vi "iRobot Navigation Display Sensors.vi"(6 "Left Wheel (mm/s)":i16, 7 "Right Wheel (mm/s)":i16, 9 "Statechart Inputs":T1={"net distance (mm)"=0, "net angle (deg)"=0, "Max Wheel Speed (mm/s)"=0, "accelerometer"={"x axis (g)"=0.0, "y axis (g)"=0.0, "z axis (g)"=0.0}, "iRobot Sensors"={"Bumps + Wheel Drops"={"Wheeldrop Caster"=FALSE, "Wheeldrop Left"=FALSE, "Wheeldrop Right"=FALSE, "Bump Left"=FALSE, "Bump Right"=FALSE}, "Wall"=FALSE, "Cliff Left"=FALSE, "Cliff Front Left"=FALSE, "Cliff Front Right"=FALSE, "Cliff Right"=FALSE, "Virtual Wall"=FALSE, "Low-Side Driver + Wheel Overcurrent"={"Low-Side Driver 0"=FALSE, "Low-Side Driver 1"=FALSE, "Low-Side Driver 2"=FALSE, "Left Wheel"=FALSE, "Right Wheel"=FALSE}, "Infrared"=255, "Buttons"={"Advance"=FALSE, "Play"=FALSE}, "Distance (mm)"=0, "Angle (deg)"=0, "Charging State"=enum."Not Charging", "Voltage (mV)"=0, "Current (mA)"=0, "Battery Temperature (deg C)"=0, "Battery Charge (mAh)"=0, "Battery Capacity (mAh)"=0, "Wall Signal (0-4095)"=0, "Cliff Left Signal (0-4095)"=0, "Cliff Front Left Signal (0-4095)"=0, "Cliff Front Right Signal (0-4095)"=0, "Cliff Right Signal (0-4095)"=0, "Cargo Bay Digital Inputs"={"Digital Input 0"=FALSE, "Digital Input 1"=FALSE, "Digital Input 2"=FALSE, "Digital Input 3"=FALSE, "Device Detect"=FALSE}, "Cargo Bay Analog Signal (0-1023)"=0, "Charging Sources Available"={"Internal Charger"=FALSE, "Home Base"=FALSE}, "OI Mode"=enum."Off", "Song Number"=0, "Song Playing"=FALSE, "Number of Stream Packets"=0, "Requested Velocity (mm/s)"=0, "Requested Radius (mm)"=0, "Requested Right Wheel Velocity (mm/s)"=0, "Requested Left Wheel Velocity (mm/s)"=0}, "Is Simulator?"=FALSE, "Edge Tape Threshold"=0, "Barcode Tape Threshold"=0, "Barcode Time Threshold"=0.0, "Barcode Action Time"=0.0, "Kp Constant"=0.0, "Ki Constant"=0.0, "Kd Constant"=0.0} {"iRobot Sensors"."Infrared" format="%02x"; "accelerometer"."z axis (g)" format="%.3f"; "accelerometer"."y axis (g)" format="%.3f"; "accelerometer"."x axis (g)" format="%.3f"; "Max Wheel Speed (mm/s)" scale=0.0..500.0}) -> (1 "iRobot Sensors (graphical)":T11 {"Right Wheel (mm/s)" scale=-500.0..500.0; "Left Wheel (mm/s)" scale=-500.0..500.0})   [LabVIEW 2015]
uses:
  iRobot Sensors.ctl
  iRobot Navigation State Machine.lvsc/Inputs.ctl
  Accelerometer.ctl
  iRobot/Sensor/Sensor Group 6.ctl
  iRobot/Sensor/Bumps + Wheel Drops.ctl
  iRobot/Sensor/Low-Side Driver + Wheel Overcurrent.ctl
  iRobot/Sensor/Buttons.ctl
  iRobot/Sensor/Charging State.ctl
  iRobot/Sensor/Cargo Bay Digital Inputs.ctl
  iRobot/Sensor/Charging Sources Available.ctl
  iRobot/Sensor/OI Mode.ctl
  iRobot Navigation State Machine.lvsc
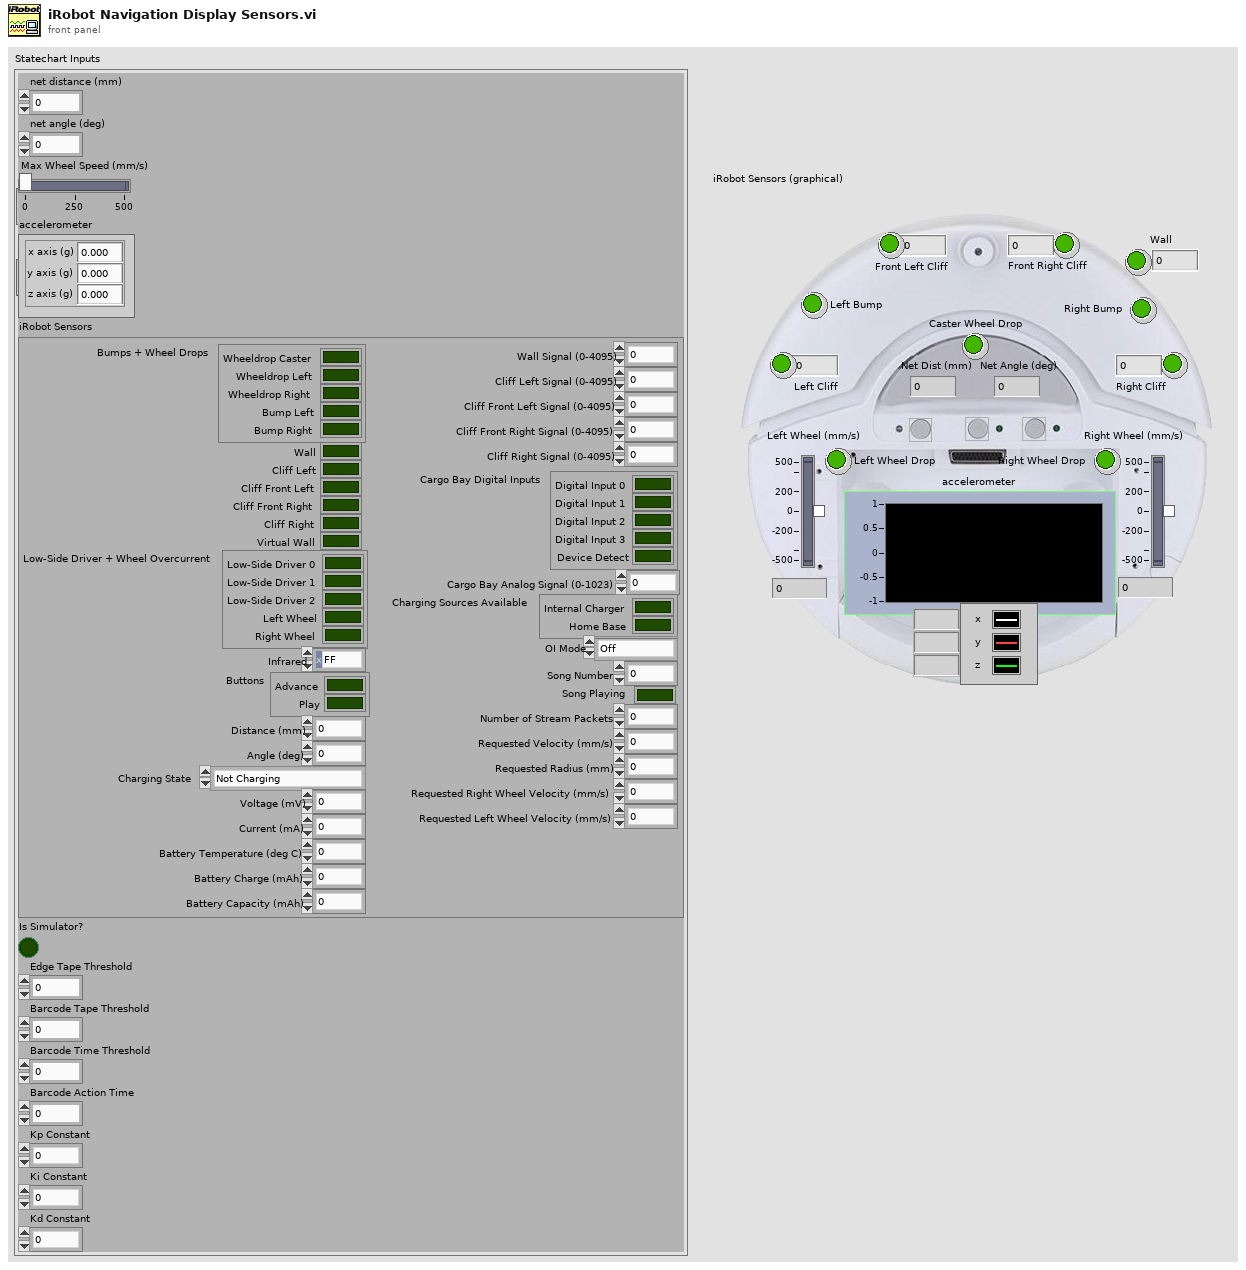
[diagram p1: front panel]
types:
  T1 = typedef "iRobot Navigation State Machine.lvsc/Inputs.ctl" = cluster{"net distance (mm)":i32, "net angle (deg)":i32, "Max Wheel Speed (mm/s)":i16, "accelerometer":T2, "iRobot Sensors":T3, "Is Simulator?":bool, "Edge Tape Threshold":u16, "Barcode Tape Threshold":u16, "Barcode Time Threshold":dbl, "Barcode Action Time":dbl, "Kp Constant":dbl, "Ki Constant":dbl, "Kd Constant":dbl}
  T2 = typedef "Accelerometer.ctl" = cluster{"x axis (g)":dbl, "y axis (g)":dbl, "z axis (g)":dbl}
  T3 = typedef "Sensor Group 6.ctl" = cluster{"Bumps + Wheel Drops":T4, "Wall":bool, "Cliff Left":bool, "Cliff Front Left":bool, "Cliff Front Right":bool, "Cliff Right":bool, "Virtual Wall":bool, "Low-Side Driver + Wheel Overcurrent":T5, "Infrared":u8, "Buttons":T6, "Distance (mm)":i32, "Angle (deg)":i32, "Charging State":T7, "Voltage (mV)":u16, "Current (mA)":i16, "Battery Temperature (deg C)":i8, "Battery Charge (mAh)":u16, "Battery Capacity (mAh)":u16, "Wall Signal (0-4095)":u16, "Cliff Left Signal (0-4095)":u16, "Cliff Front Left Signal (0-4095)":u16, "Cliff Front Right Signal (0-4095)":u16, "Cliff Right Signal (0-4095)":u16, "Cargo Bay Digital Inputs":T8, "Cargo Bay Analog Signal (0-1023)":u16, "Charging Sources Available":T9, "OI Mode":T10, "Song Number":u8, "Song Playing":bool, "Number of Stream Packets":u8, "Requested Velocity (mm/s)":i16, "Requested Radius (mm)":i16, "Requested Right Wheel Velocity (mm/s)":i16, "Requested Left Wheel Velocity (mm/s)":i16}
  T4 = typedef "Bumps + Wheel Drops.ctl" = cluster{"Wheeldrop Caster":bool, "Wheeldrop Left":bool, "Wheeldrop Right":bool, "Bump Left":bool, "Bump Right":bool}
  T5 = typedef "Low-Side Driver + Wheel Overcurrent.ctl" = cluster{"Low-Side Driver 0":bool, "Low-Side Driver 1":bool, "Low-Side Driver 2":bool, "Left Wheel":bool, "Right Wheel":bool}
  T6 = typedef "Buttons.ctl" = cluster{"Advance":bool, "Play":bool}
  T7 = typedef "Charging State.ctl" = enum16{"Not Charging", "Reconditioning Charging", "Full Charging", "Trickle Charging", "Waiting", "Charging Fault Condition"}
  T8 = typedef "Cargo Bay Digital Inputs.ctl" = cluster{"Digital Input 0":bool, "Digital Input 1":bool, "Digital Input 2":bool, "Digital Input 3":bool, "Device Detect":bool}
  T9 = typedef "Charging Sources Available.ctl" = cluster{"Internal Charger":bool, "Home Base":bool}
  T10 = typedef "OI Mode.ctl" = enum16{"Off", "Passive", "Safe", "Full"}
  T11 = typedef "iRobot Sensors.ctl" = cluster{"Caster Wheel Drop":bool, "Left Wheel Drop":bool, "Right Wheel Drop":bool, "Left Bump":bool, "Right Bump":bool, "Left Cliff":bool, "Front Left Cliff":bool, "Front Right Cliff":bool, "Right Cliff":bool, "Wall":bool, "Net Dist (mm)":i32, "Net Angle (deg)":i32, "Wall":u16, "Left Cliff":u16, "Front Left Cliff":u16, "Front Right Cliff":u16, "Right Cliff":u16, "Left Wheel (mm/s)":i16, "Right Wheel (mm/s)":i16, "accelerometer":T2}
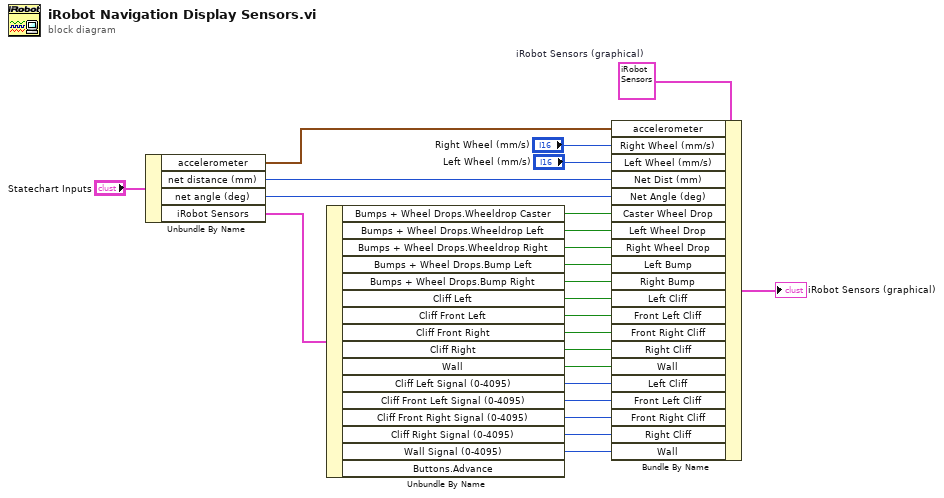
[diagram p0: block diagram]
diagram:
  w7 = T11 {"Caster Wheel Drop"=FALSE, "Left Wheel Drop"=FALSE, "Right Wheel Drop"=FALSE, "Left Bump"=FALSE, "Right Bump"=FALSE, "Left Cliff"=FALSE, "Front Left Cliff"=FALSE, "Front Right Cliff"=FALSE, "Right Cliff"=FALSE, "Wall"=FALSE, "Net Dist (mm)"=0, "Net Angle (deg)"=0, "Wall"=0, "Left Cliff"=0, "Front Left Cliff"=0, "Front Right Cliff"=0, "Right Cliff"=0, "Left Wheel (mm/s)"=0, "Right Wheel (mm/s)"=0, "accelerometer"={"x axis (g)"=0.0, "y axis (g)"=0.0, "z axis (g)"=0.0}}  # iRobot Sensors (graphical)
  n1 = Unbundle By Name("Statechart Inputs") -> ("accelerometer"=w2:T2, "net distance (mm)"=w3:i32, "net angle (deg)"=w4:i32, "iRobot Sensors"=w5:T3)
  n2 = Unbundle By Name(w5) -> ("Bumps + Wheel Drops.Wheeldrop Caster"=w24:bool, "Bumps + Wheel Drops.Wheeldrop Left"=w23:bool, "Bumps + Wheel Drops.Wheeldrop Right"=w22:bool, "Bumps + Wheel Drops.Bump Left"=w21:bool, "Bumps + Wheel Drops.Bump Right"=w20:bool, "Cliff Left"=w19:bool, "Cliff Front Left"=w18:bool, "Cliff Front Right"=w17:bool, "Cliff Right"=w16:bool, "Wall"=w15:bool, "Cliff Left Signal (0-4095)"=w14:u16, "Cliff Front Left Signal (0-4095)"=w13:u16, "Cliff Front Right Signal (0-4095)"=w12:u16, "Cliff Right Signal (0-4095)"=w11:u16, "Wall Signal (0-4095)"=w10:u16)  [unwired: 1 out]
  n3 = Bundle By Name(cluster=w7, "accelerometer"=w2, "Right Wheel (mm/s)"="Right Wheel (mm/s)", "Left Wheel (mm/s)"="Left Wheel (mm/s)", "Net Dist (mm)"=w3, "Net Angle (deg)"=w4, "Caster Wheel Drop"=w24, "Left Wheel Drop"=w23, "Right Wheel Drop"=w22, "Left Bump"=w21, "Right Bump"=w20, "Left Cliff"=w19, "Front Left Cliff"=w18, "Front Right Cliff"=w17, "Right Cliff"=w16, "Wall"=w15, "Left Cliff"=w14, "Front Left Cliff"=w13, "Front Right Cliff"=w12, "Right Cliff"=w11, "Wall"=w10) -> (→"iRobot Sensors (graphical)":T11)
